vi "insertData.vi"(7 "db_File":path=path "C:/Users/YuanYuan/Desktop/Labview Data/Database", 8 "P":dbl[](array[numeric]), 9 "Z":dbl[](array[numeric]), 10 "frequency":dbl[](array[numeric]), 11 "exp_ID":i32) -> (0 "error out":errorcluster)   [LabVIEW 2014, in "ChirpV2.lvclass"]
doc: "This example allows you to perform several tasks on the specified table in a database named LabVIEW.mdb located in the LabVIEW examples>>database directory.\n\nThis VI is running when you open it. Select one of the tabs and enter the appropriate data. Press the Go button to complete the displayed tab option.\n\nAutomatic - This option inserts a new record into the specified table. The record is specified by a cluster containing the correct number of elements and of the data types defined by the specified table. \n\nSQL Query - This option performs the specified SQL query.\n\nParameterized SQL Query - This option performs the specified SQL query as a parameterized SQL Query. This method is faster and more efficient than directly executing an SQL query because it sets up all the parameters prior to doing the command."
uses:
  EIS/Electrochemical Instrument Folder/Chirp_OOP/ChirpV2.lvclass
  <vilib>/addons/database/Connection.llb/DB Tools Open Connec (String).vi
  <vilib>/addons/database/NI_Database_API.lvlib
panel:
  # "Overview: Demonstrates how to insert records into databases, and perform SQL queries.\nRequirements: Database Connectivity Toolkit\nInstructions:\nRun the VI."
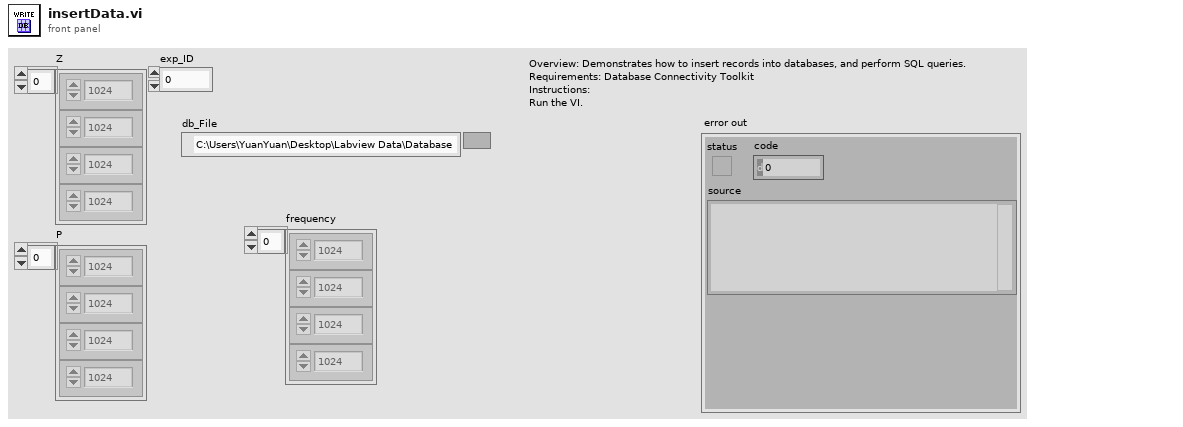
[diagram p1: front panel]
types:
  T1 = typedef "NI_Database_API.lvlib/Conn ObjectReference.ctl" = refnum<k1>
  T2 = cluster{"exp_ID":i32, "frequency":dbl, "Z":dbl, "P":dbl}
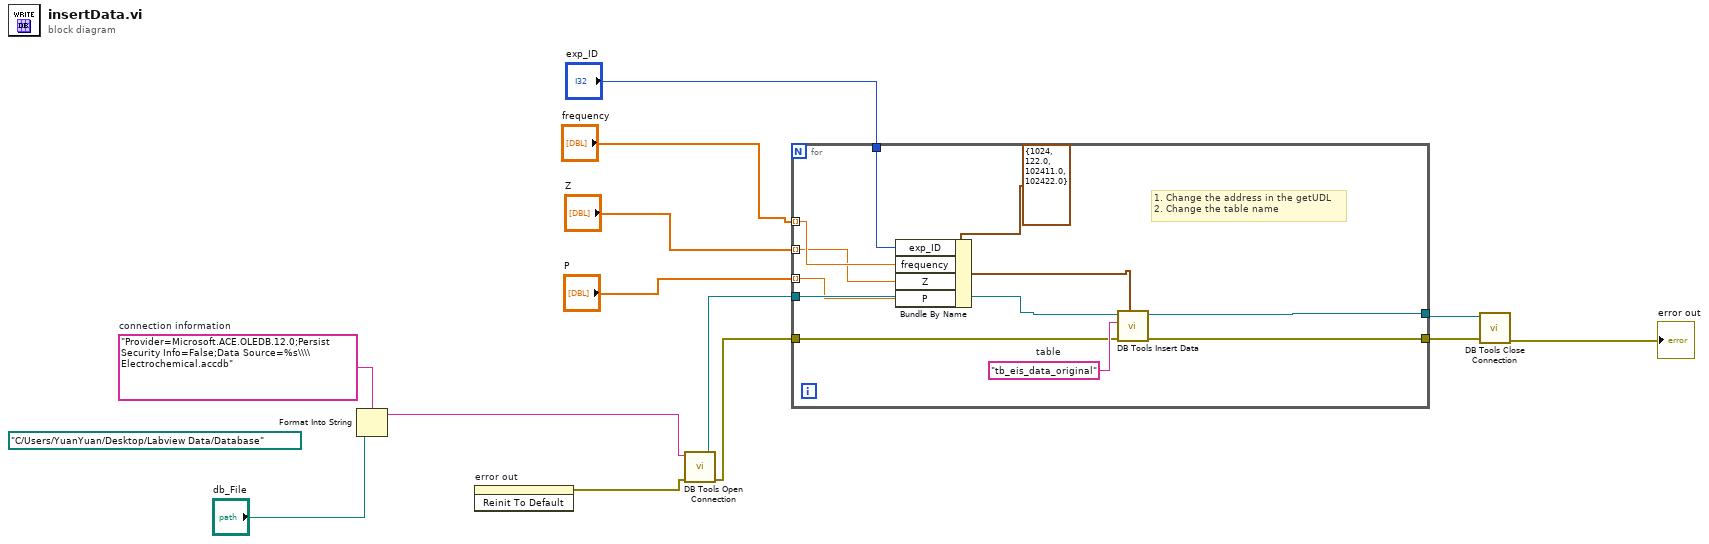
[diagram p0: block diagram]
diagram:
  (unwired) path "C:/Users/YuanYuan/Desktop/Labview Data/Database" ("path")
  w6 = "Provider=Microsoft.ACE.OLEDB.12.0;Persist Security Info=False;Data Source=%s\\\\Electrochemical.accdb"  # connection information
  n1 = Format Into String(format string=w6, "db_File") -> (resulting string=w4:string)  [unwired: 2 in, 1 out]
  n2 = invoke on="error out" class="Clust (strict)" method="Reinit To Default"() -> (error out=w7:errorcluster)  [unwired: 3 in, 2 out]
  n3 = call-poly <vilib>:"DB Tools Open Connection.vi"("error in (no error)"=w7, "connection information"=w4) -> ("error out"=w11:errorcluster, "connection reference"=w12:T1)  [unwired: 6 in]
  n4 = for {
    tunnel: "frequency" -> [w17] mode=indexing
    tunnel: w12 -> [w21]
    tunnel: w11 -> [w20]
    tunnel: [w19] -> w10
    tunnel: [w18] -> w9
    tunnel: "Z" -> [w16] mode=indexing
    tunnel: "P" -> [w15] mode=indexing
    tunnel: "exp_ID" -> [w14]
    w24 = "tb_eis_data_original"  # table
    # "1. Change the address in the getUDL\n2. Change the table name"
    n5 = Bundle By Name(cluster=T2 {"exp_ID"=1024, "frequency"=122.0, "Z"=102411.0, "P"=102422.0} ("Data"), "exp_ID"=w14, "frequency"=w17, "Z"=w16, "P"=w15) -> (w22:T2)
    n6 = call <vilib>:"DB Tools Insert Data.vi"("data"=w22, "error in (no error)"=w20, "table"=w24, "connection reference"=w21) -> ("error out"=w18:errorcluster, "connection reference out"=w19:T1)  [unwired: 6 in]
  }
  n7 = call <vilib>:"DB Tools Close Connection.vi"("error in (no error)"=w9, "connection reference"=w10) -> ("error out"=→"error out":errorcluster)  [unwired: 5 in]
